vi "Ctor.vi"(8 "error in (no error)":errorcluster, 11 "Name":string) -> (0 "error out":errorcluster, 3 "Chat Client out":refnum<class "Chat Client.lvclass">)   [LabVIEW 2020, in "Chat Client.lvclass"]
uses:
  Chat Client.lvclass
  Stream-TCP/TCP Client/TCP Client.lvclass
  C:/Program Files (x86)/National Instruments/LabVIEW 2020/vi.lib/IlluminatedG/lv-stream/Endpoint/Endpoint.lvclass
  Chat Client.lvclass/Chat Client.ctl
  <vilib>/IlluminatedG/lv-stream/Endpoint/Endpoint.lvclass
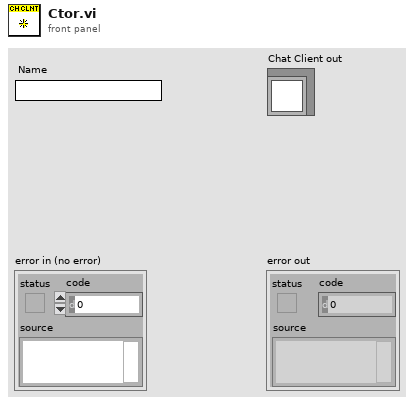
[diagram p1: front panel]
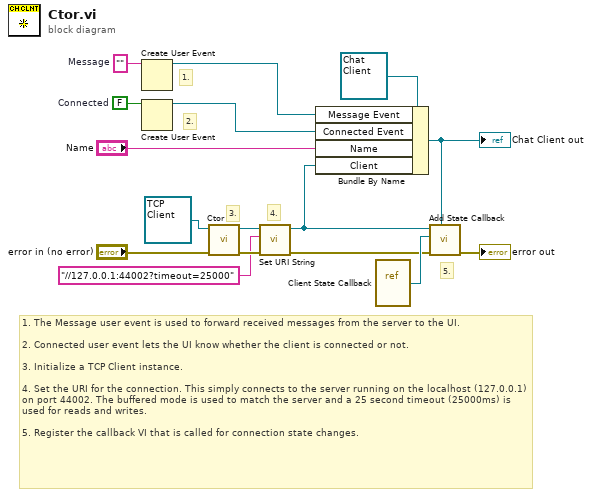
[diagram p0: block diagram]
diagram:
  w5 = ""  # Message
  w9 = FALSE  # Connected
  # "1. The Message user event is used to forward received messages from the server to the UI.\n\n2. Connected user event lets the UI know whether the client is connected or not.\n\n3. Initialize a TCP Client instance.\n\n4. Set the URI for the connection. This simply connects to the server running on the localhost (127.0.0.1) on port 44002. The buffered mode is used to match the server and a 25 second timeout (25000ms) is used for reads and writes.\n\n5. Register the callback VI that is called for connection state changes."
  # "5."
  # "4."
  # "3."
  # "2."
  # "1."
  n1 = Create User Event(user event datatype=w5) -> (user event=w4:refnum<user-event>)  [unwired: 1 in, 1 out]
  n2 = Create User Event(user event datatype=w9) -> (user event=w8:refnum<user-event>)  [unwired: 1 in, 1 out]
  n3 = call-dynamic "Ctor.vi"("error in (no error)"="error in (no error)", "TCP Client in"=refnum<class "TCP Client.lvclass"> refnum) -> ("error out"=w16:errorcluster, "TCP Client out"=w13:refnum<class "TCP Client.lvclass">)  [unwired: 8 in]
  n4 = call <vilib>:"Set URI String.vi"("error in (no error)"=w16, "URI String"="//127.0.0.1:44002?timeout=25000", "Endpoint in"=w13) -> ("error out"=w2:errorcluster, "Endpoint out"=w10:refnum<class "TCP Client.lvclass">)  [unwired: 7 in]
  n5 = Bundle By Name(cluster=refnum<class "Chat Client.lvclass"> refnum ("Chat Client in"), "Message Event"=w4, "Connected Event"=w8, "Name"="Name", "Client"=w10) -> (w7:refnum<class "Chat Client.lvclass">)
  "Chat Client out" <- w7
  n6 = vi-ref "Client State Callback.vi"() -> (w6:refnum<vi>)
  n7 = call-dynamic "Add State Callback.vi"("Owner (None)"=w7, "error in (no error)"=w2, "Callback"=w6, "Connection in"=w10) -> ("error out"=→"error out":errorcluster)  [unwired: 6 in, 1 out]
